vi "practica8_grafica.vi"() -> ()   [LabVIEW 2013]
panel:
  out "fecha y hora":string
  in  "rango de muestreo (ms)":u32
  in  "limite superior":dbl
  in  "puntos a adquirir":dbl
  out "puntos adquiridos":i32
  in  "stop":bool
  out "fuera de rango":bool
  out "temperatura":cluster{dbl, "limite superior":dbl}(graph)
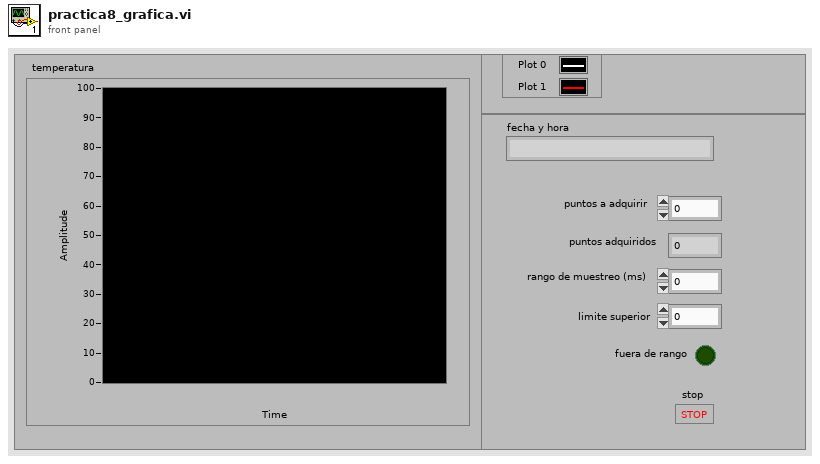
[diagram p1: front panel]
types:
  T1 = cluster{"number: 0 to 1":dbl, "limite superior":dbl}[]
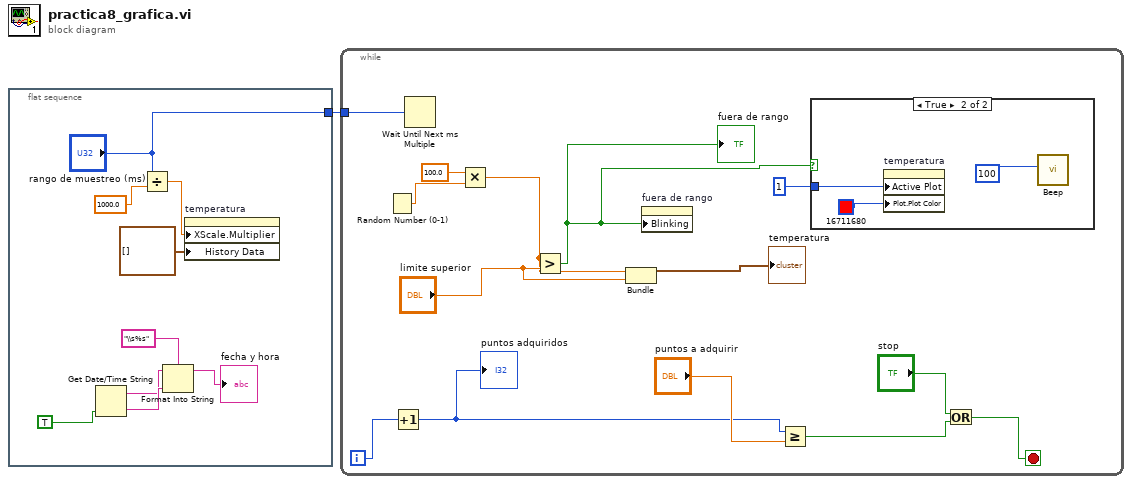
[diagram p0: block diagram]
diagram:
  n1 = flat-sequence {
    tunnel: ["rango de muestreo (ms)"] -> w1
    frame #0 {
      n2 = Get Date/Time String(want seconds? (F)=TRUE) -> (date string=w4:string, time string=w5:string)  [unwired: 2 in]
      n3 = Divide(x="rango de muestreo (ms)", y=1000.0) -> (x/y=w9:dbl)
      n4 = Format Into String(format string="\\s%s", initial string=w4, w5) -> (resulting string=→"fecha y hora":string)  [unwired: 1 in, 1 out]
      n5 = property on="temperatura" class="WFChart (strict)"("XScale.Multiplier"=w9, "History Data"=T1 []) -> ()  [unwired: 2 in, 2 out]
    }
  }
  n6 = while {
    tunnel: w1 -> [w14]
    i -> [w21]
    stop <- w24 stop-if-true
    n7 = Random Number (0-1)() -> (number: 0 to 1=w13:dbl)
    n8 = Increment(x=w21) -> (x+1=w19:i32)
    "puntos adquiridos" <- w19
    n9 = Wait Until Next ms Multiple(millisecond multiple=w14) -> ()  [unwired: 1 out]
    n10 = Multiply(x=100.0, y=w13) -> (x*y=w11:dbl)
    n11 = Greater?(x=w11, y="limite superior") -> (0:w16:bool)
    "fuera de rango" <- w16
    n12 = Bundle(w11, "limite superior"="limite superior") -> (→"temperatura":cluster{dbl, "limite superior":dbl})  [unwired: 1 in]
    n13 = property on="fuera de rango" class="Bool (strict)"("Blinking"=w16) -> ()  [unwired: 2 in, 2 out]
    n14 = Greater Or Equal?(x=w19, y="puntos a adquirir") -> (x >= y?=w22:bool)
    n15 = case shown="True" w16 {
      tunnel: u32 1 ("Active Plot") -> [_ w27]
      frame False {
      }
      frame True {
        n16 = property on="temperatura" class="WFChart (strict)"("Active Plot"=w27, "Plot.Plot Color"=u32 16711680) -> ()  [unwired: 2 in, 2 out]
        n17 = call <vilib>:"Beep.vi"("duration (msec)"=u32 100) -> ()  [unwired: 11 in]
      }
    }
    n18 = Or(x="stop", y=w22) -> (x .or. y?=w24:bool)
  }
